vi "Updata NodePath.vi"(8 "error in":errorcluster caption="错误输入（无错误）", 10 "Parent Path":string, 11 "PanelLinkNode 输入":refnum<class "PanelLinkNode.lvclass"> caption="DNL_LabVIEW Object in") -> (0 "error out":errorcluster caption="错误输出", 3 "PanelLinkNode 输出":refnum<class "PanelLinkNode.lvclass"> caption="DNL_LabVIEW Object out")   [LabVIEW 2013, in "PanelLinkNode.lvclass"]
uses:
  PanelLinkNode.lvclass
  PanelLinkNode.lvclass/PanelLinkNode.ctl
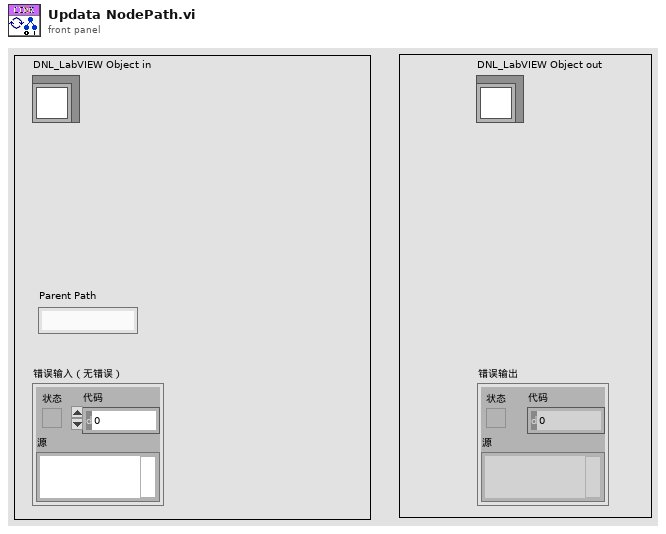
[diagram p1: front panel]
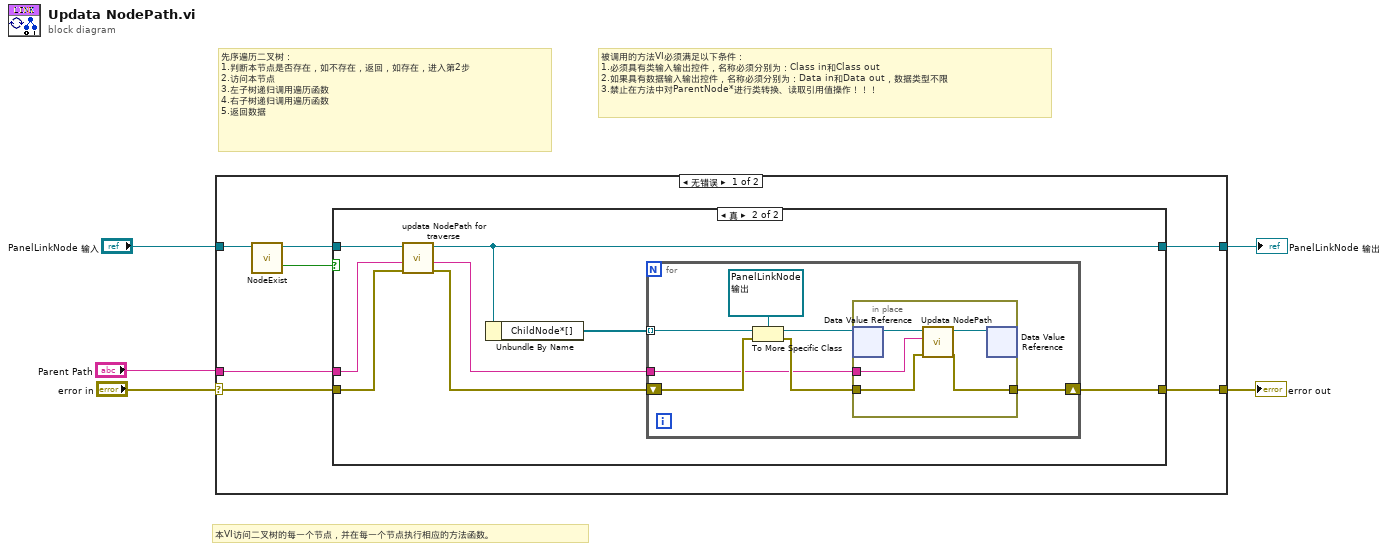
[diagram p0: block diagram]
diagram:
  # "本VI访问二叉树的每一个节点，并在每一个节点执行相应的方法函数。"
  # "被调用的方法VI必须满足以下条件：\n1.必须具有类输入输出控件，名称必须分别为：Class in和Class out\n2.如果具有数据输入输出控件，名称必须分别为：Data in和Data out，数据类型不限\n3.禁止在方法中对ParentNode*进行类转换、读取引用值操作！！！"
  # "先序遍历二叉树：\n1.判断本节点是否存在，如不存在，返回，如存在，进入第2步\n2.访问本节点\n3.左子树递归调用遍历函数\n4.右子树递归调用遍历函数\n5.返回数据"
  n1 = case shown="无错误" "error in" {
    selector: "error in" -> [w7 w36]
    tunnel: [w8 w36] -> w4
    tunnel: [w12 w35] -> w2
    tunnel: "PanelLinkNode 输入" -> [w10 w35]
    tunnel: "Parent Path" -> [w11 _]
    frame No Error {
      n2 = call-dynamic "NodeExist.vi"("PanelLinkNode 输入"=w10) -> ("Node Exist?"=w6:bool, "PanelLinkNode 输出"=w9:refnum<class "PanelLinkNode.lvclass">)  [unwired: 8 in, 1 out]
      n3 = case shown="真" w6 {
        tunnel: [w14 w19] -> w12
        tunnel: w11 -> [_ w16]
        tunnel: w9 -> [w14 w20]
        tunnel: [w13 w21] -> w8
        tunnel: w7 -> [w13 w18]
        frame False {
        }
        frame True {
          n4 = call-dynamic "updata NodePath for traverse.vi"("error in (no error)"=w18, "Data in"=w16, "Class in"=w20) -> ("error out"=w17:errorcluster, "Data out"=w15:string, "Class out"=w19:refnum<class "PanelLinkNode.lvclass">)  [unwired: 6 in]
          n5 = Unbundle By Name(w19) -> ("ChildNode*[]"=w22:refnum<data-value>[])
          n6 = for {
            tunnel: w22 -> [w28] mode=indexing
            shift-right: [w25] -> w21
            shift-left: w17 -> [w24]
            tunnel: w15 -> [w23]
            n7 = To More Specific Class(target class=refnum<data-value> refnum ("数据值引用"), reference=w28, error in=w24) -> (specific class reference=w27:refnum<data-value>, error out=w26:errorcluster)
            n8 = in-place {
              in-place-border: w23 -> [w32]
              in-place-border: w26 -> [w31]
              in-place-border: [w30] -> w25
              n9 = in-place-dvr #1(w27) -> (w34:refnum<class "PanelLinkNode.lvclass">)  [unwired: 1 out]
              n10 = call-dynamic "Updata NodePath.vi"("error in"=w31, "Parent Path"=w32, "PanelLinkNode 输入"=w34) -> ("error out"=w30:errorcluster, "PanelLinkNode 输出"=w33:refnum<class "PanelLinkNode.lvclass">)  [unwired: 7 in]
              n11 = in-place-dvr #1(w33) -> ()  [unwired: 2 out]
            }
          }
        }
      }
    }
    frame Error {
    }
  }
  "error out" <- w4
  "PanelLinkNode 输出" <- w2
